vi "LVObject to JSON.vi"(8 "error in (no error)":errorcluster, 11 "LabVIEW Object in":refnum<class>) -> (0 "error out":errorcluster, 3 "<JSON>":string)   [LabVIEW 2019, in "JSONtext.lvlib"]
uses:
  JSONtext.lvlib
  Base64/Base64 Support.lvlib
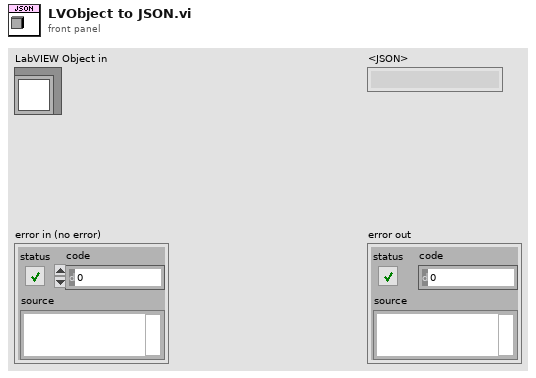
[diagram p1: front panel]
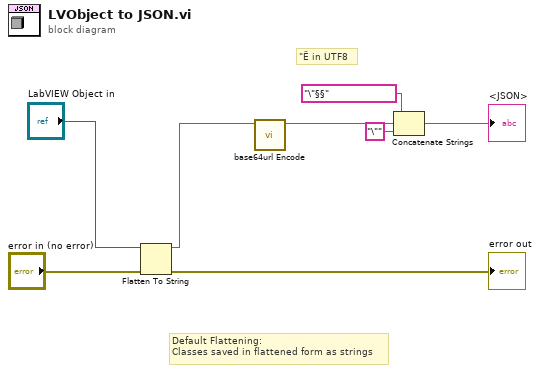
[diagram p0: block diagram]
diagram:
  # "\"Ё in UTF8"
  # "Default Flattening:\nClasses saved in flattened form as strings"
  n1 = Flatten To String(anything="LabVIEW Object in", error in (no error)="error in (no error)") -> (data string=w5:string, error out=→"error out":errorcluster)  [unwired: 2 in, 1 out]
  n2 = call "base64url Encode.vi"("String"=w5) -> ("base64url"=w4:string)  [unwired: 10 in]
  n3 = Concatenate Strings("\"§§" ("string"), w4, "\"" ("string")) -> (→"<JSON>":string)
